vi "Find_Number_Line.vi"(3 "error in":errorcluster, 4 "Test Paragraph":string, 5 "Row Headers[]":string[](array[string])) -> (0 "error out":errorcluster, 1 "1 line Test ?":bool, 2 "Line number":i32)   [LabVIEW 2017]
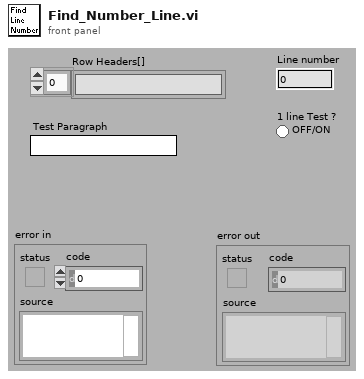
[diagram p1: front panel]
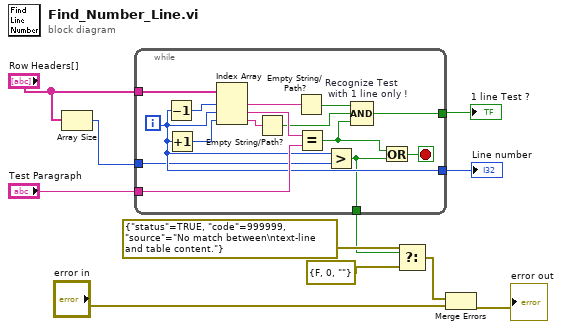
[diagram p0: block diagram]
diagram:
  n1 = Array Size(array="Row Headers[]") -> (size(s)=w7:i32)
  n2 = while {
    tunnel: "Test Paragraph" -> [w26]
    tunnel: "Row Headers[]" -> [w25]
    tunnel: [w16] -> w10
    tunnel: [w15] -> w11
    tunnel: w7 -> [w14]
    tunnel: [w13] -> w3
    i -> [w15]
    stop <- w17 stop-if-true
    n3 = Decrement(x=w15) -> (x-1=w24:i32)
    n4 = Increment(x=w15) -> (x+1=w23:i32)
    n5 = Index Array(array=w25, index #1=w24, index #2=w15, index #3=w23) -> (element #1=w21:string, element #2=w22:string, element #3=w20:string)
    n6 = Empty String/Path?(string/path=w20) -> (empty?=w18:bool)
    n7 = Empty String/Path?(string/path=w21) -> (empty?=w19:bool)
    n8 = Equal?(x=w22, y=w26) -> (x = y?=w12:bool)
    n9 = Greater?(x=w15, y=w14) -> (0:w13:bool)
    n10 = Compound Arithmetic op=AND "Recognize Test \n with 1 line only !"(w19, w18, w12) -> (w16:bool)
    n11 = Or(x=w12, y=w13) -> (x .or. y?=w17:bool)
  }
  "Line number" <- w11
  "1 line Test ?" <- w10
  n12 = Select(t=errorcluster {"status"=TRUE, "code"=999999, "source"="No match between\ntext-line and table content."} ("error in 1 (no error)"), s=w3, f=errorcluster {"status"=FALSE, "code"=0, "source"=""}) -> (s? t:f=w1:errorcluster)
  n13 = Merge Errors(w1, "error in") -> (→"error out":errorcluster)
